vi "CheckWavelengthGrating.vi"(7 "Monochromator in":T1={"Type"=enum."PTI", "Wavelength (nm)"=600.0, "Grating, gr/mm"=enum."1200", "Grating mode"=enum."Visible", "Spectrum mode"={"Spectrum mode?"=FALSE, "Start wavelength (nm)"=0.0, "End wavelength (nm)"=0.0, "Wavelength step (nm)"=0.0, "Wavelength array"=[], "array index"=0}, "PTI"={"Delay before read (ms)"=300, "Mono 1"={"Timeout (ms)"=1000, "Resource Name"="COM5", "Baud Rate"=9600, "Data Bits"=8, "Parity"=0, "Stop Bits"=10, "Flow Control"=0}, "Mono 2"={"Timeout (ms)"=1000, "Resource Name"="COM6", "Baud Rate"=9600, "Data Bits"=8, "Parity"=0, "Stop Bits"=10, "Flow Control"=0}, "Two PTI Monochromators?"=FALSE}, "Oriel (custom)"={"reference"=refnum}, "Force wavelength confirmation (PTI)?"=FALSE} {"PTI"."Mono 2"."Flow Control" items=["1.0"=10, "1.5"=15, "2.0"=20]; "PTI"."Mono 2"."Stop Bits" items=["None", "Odd", "Even", "Mark", "Space"]; "PTI"."Mono 2"."Parity" items=["None", "Odd", "Even", "Mark", "Space"]; "PTI"."Mono 1"."Flow Control" items=["1.0"=10, "1.5"=15, "2.0"=20]; "PTI"."Mono 1"."Stop Bits" items=["None", "Odd", "Even", "Mark", "Space"]; "PTI"."Mono 1"."Parity" items=["None", "Odd", "Even", "Mark", "Space"]}, 8 "error in (no error)":errorcluster, 10 "Enable wavelength input? (F)":bool, 11 "Wavelength (nm)":dbl=600.0) -> (0 "error out":errorcluster, 5 "Monochromator out":T1={"Type"=enum."PTI", "Wavelength (nm)"=600.0, "Grating, gr/mm"=enum."1200", "Grating mode"=enum."Visible", "Spectrum mode"={"Spectrum mode?"=FALSE, "Start wavelength (nm)"=0.0, "End wavelength (nm)"=0.0, "Wavelength step (nm)"=0.0, "Wavelength array"=[], "array index"=0}, "PTI"={"Delay before read (ms)"=300, "Mono 1"={"Timeout (ms)"=1000, "Resource Name"="COM5", "Baud Rate"=9600, "Data Bits"=8, "Parity"=0, "Stop Bits"=10, "Flow Control"=0}, "Mono 2"={"Timeout (ms)"=1000, "Resource Name"="COM6", "Baud Rate"=9600, "Data Bits"=8, "Parity"=0, "Stop Bits"=10, "Flow Control"=0}, "Two PTI Monochromators?"=FALSE}, "Oriel (custom)"={"reference"=refnum}, "Force wavelength confirmation (PTI)?"=FALSE} {"PTI"."Mono 2"."Flow Control" items=["1.0"=10, "1.5"=15, "2.0"=20]; "PTI"."Mono 2"."Stop Bits" items=["None", "Odd", "Even", "Mark", "Space"]; "PTI"."Mono 2"."Parity" items=["None", "Odd", "Even", "Mark", "Space"]; "PTI"."Mono 1"."Flow Control" items=["1.0"=10, "1.5"=15, "2.0"=20]; "PTI"."Mono 1"."Stop Bits" items=["None", "Odd", "Even", "Mark", "Space"]; "PTI"."Mono 1"."Parity" items=["None", "Odd", "Even", "Mark", "Space"]})   [LabVIEW 2017, in "Monochromator.lvlib" / "PTI.lvlib"]
uses:
  PTI.lvlib
  Controls/Params.ctl
  Controls/Type.ctl
  Controls/GratingValues.ctl
  Controls/Grating.ctl
  Controls/VISA parameters.ctl
  Custom Oriel drivers/Controls/Params.ctl
  C:/Project Work/icl-optical-software-rewrite/Optical Software Code Simplified/Modules/Monochromator/Cornerstone.dll
  Cornerstone.dll
  Monochromator.lvlib
  Serial comms/Serial comms.lvlib
  Custom Oriel drivers/Oriel (custom drivers).lvlib
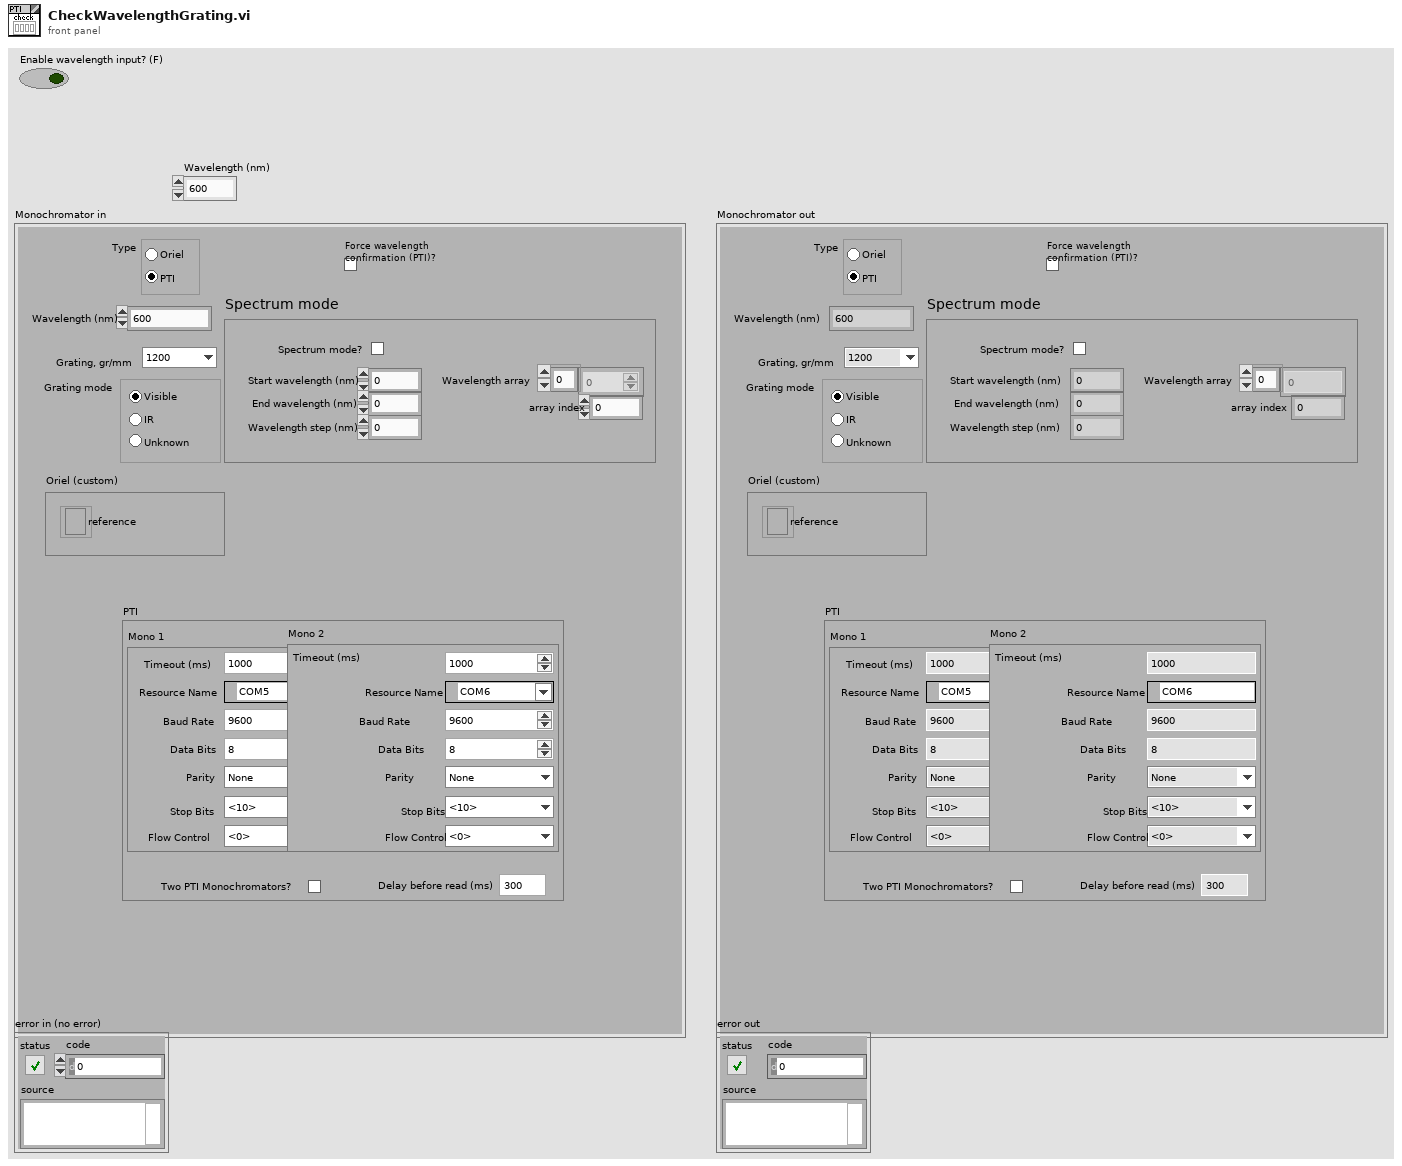
[diagram p1: front panel]
types:
  T1 = typedef "Monochromator.lvlib/Params.ctl" = cluster{"Type":T2, "Wavelength (nm)":dbl, "Grating, gr/mm":T3, "Grating mode":T4, "Spectrum mode":cluster{"Spectrum mode?":bool, "Start wavelength (nm)":dbl, "End wavelength (nm)":dbl, "Wavelength step (nm)":dbl, "Wavelength array":dbl[], "array index":u32}, "PTI":T5, "Oriel (custom)":T7, "Force wavelength confirmation (PTI)?":bool}
  T2 = typedef "Monochromator.lvlib/Type.ctl" = enum32{"Oriel", "PTI"}
  T3 = typedef "Monochromator.lvlib/GratingValues.ctl" = enum16{"2400", "1800", "1200", "600", "300", "150"}
  T4 = typedef "Monochromator.lvlib/Grating.ctl" = enum32{"Unknown", "Visible", "IR"}
  T5 = typedef "Monochromator.lvlib/PTI.lvlib/Params.ctl" = cluster{"Delay before read (ms)":u32, "Mono 1":T6, "Mono 2":T6, "Two PTI Monochromators?":bool}
  T6 = typedef "Serial comms.lvlib/VISA parameters.ctl" = cluster{"Timeout (ms)":u32, "Resource Name":refnum<visa-resource-name>, "Baud Rate":u32, "Data Bits":u16, "Parity":u16, "Stop Bits":u16, "Flow Control":u16}
  T7 = typedef "Monochromator.lvlib/Oriel (custom drivers).lvlib/Params.ctl" = cluster{"reference":refnum<k24>}
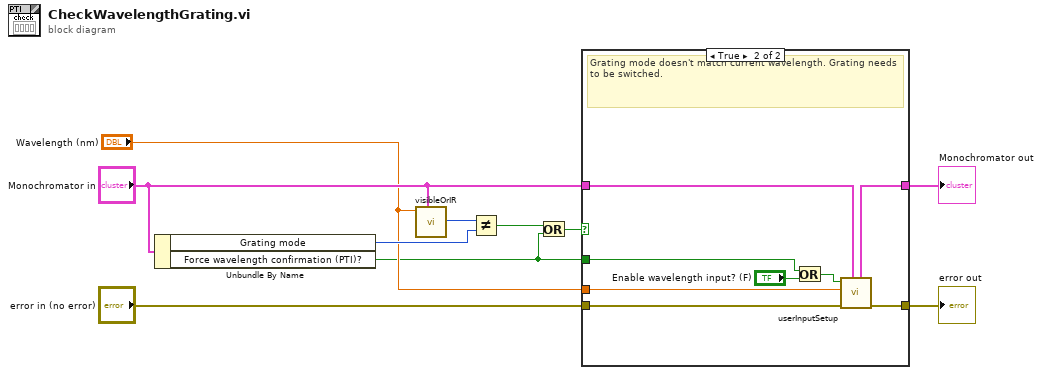
[diagram p0: block diagram]
diagram:
  n1 = Unbundle By Name("Monochromator in") -> ("Grating mode"=w10:T4, "Force wavelength confirmation (PTI)?"=w1:bool)
  n2 = call "visibleOrIR.vi"("Monochromator"="Monochromator in", "Wavelength (nm)"="Wavelength (nm)") -> ("IR/visible"=w9:T4)  [unwired: 7 in, 2 out]
  n3 = Not Equal?(x=w9, y=w10) -> (x != y?=w2:bool)
  n4 = Or(x=w2, y=w1) -> (x .or. y?=w3:bool)
  n5 = case shown="True" w3 {
    tunnel: "error in (no error)" -> [w12 w20]
    tunnel: [w12 w19] -> w6
    tunnel: [w11 w18] -> w7
    tunnel: "Monochromator in" -> [w11 w17]
    tunnel: "Wavelength (nm)" -> [_ w16]
    tunnel: w1 -> [_ w13]
    frame False {
      # "Wavelength and grating match."
    }
    frame True {
      # "Grating mode doesn't match current wavelength. Grating needs to be switched."
      n6 = Or(x=w13, y="Enable wavelength input? (F)") -> (x .or. y?=w15:bool)
      n7 = call "userInputSetup.vi"("Monochromator"=w17, "error in (no error)"=w20, "Wavelength (nm)"=w16, "Enable wavelength input?"=w15) -> ("error out"=w19:errorcluster, "Monochromator out"=w18:T1)  [unwired: 6 in]
    }
  }
  "Monochromator out" <- w7
  "error out" <- w6
